vi "Create URI.vi"(0 "IP Address":string, 2 "Port (80)":u16=80, 4 "Service Name":string) -> (16 "URI":string)   [LabVIEW 2017, in "LV WebSockets.lvlib"]
doc: "Create a valid websocket URI staring form IP address, port and service name. THis VI is intended to facilitate the code modifications required when upgrading form older versions of the library where the the client handshake VI was not taking a ws URI as input but IP address and port separately"
uses:
  LV WebSockets.lvlib
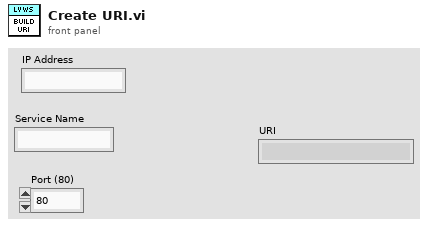
[diagram p1: front panel]
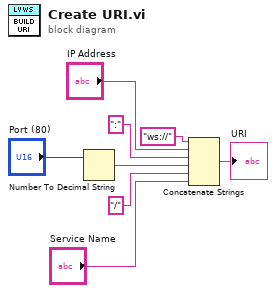
[diagram p0: block diagram]
diagram:
  n1 = Number To Decimal String(number="Port (80)") -> (decimal integer string=w4:string)  [unwired: 1 in]
  n2 = Concatenate Strings("ws://" ("string"), "IP Address", ":" ("string"), w4, "/" ("string"), "Service Name") -> (→"URI":string)
